vi "test report.vi"(6 "append report?":bool=TRUE, 7 "report path":path=path "C:/Users/andreika/Documents/work/SPELS_TEST/stm_test/TestReport.xlsx", 8 "error in":errorcluster, 9 "MS Office parameters in":T1, 10 "report in":refnum<class "NI_report.lvclass">, 11 "test data cluster":T2 {"elements 2" format="%x"; "elements 1" format="%x"}) -> (0 "error out":errorcluster, 1 "report path out":path, 2 "MS Office parameters out":T1, 3 "report out":refnum<class "NI_report.lvclass">)   [LabVIEW 2017, in "SPELS test.lvlib"]
uses:
  SPELS test.lvlib
  <vilib>/Utility/NIReport.llb/NI_report.lvclass
  <vilib>/Utility/NIReport.llb/Append Report Text (str wrap).vi
  <vilib>/Utility/NIReport.llb/Excel/NI_Excel.lvclass
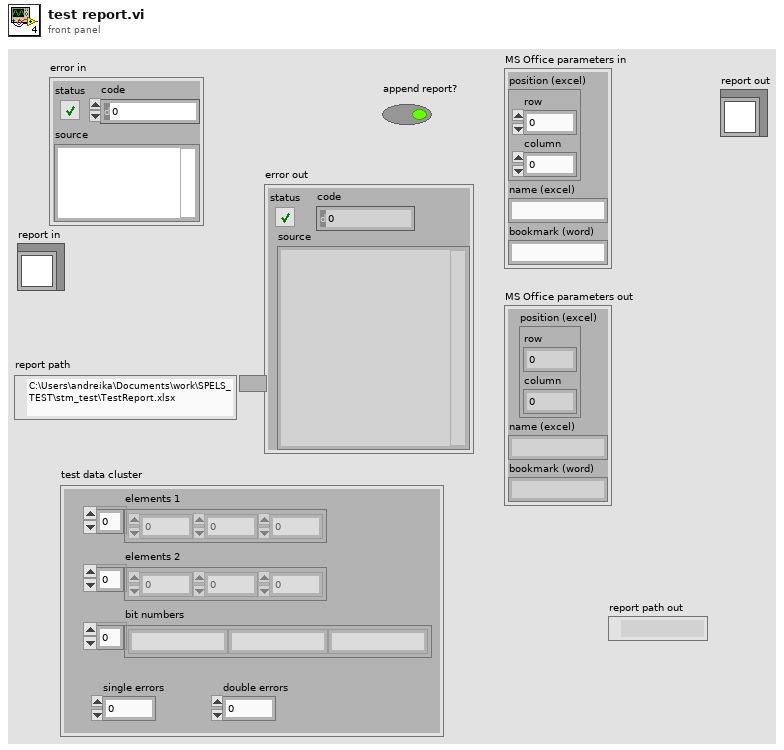
[diagram p1: front panel]
types:
  T1 = cluster{"position (excel)":cluster{"row":i32, "column":i32}, "name (excel)":string, "bookmark (word)":string}
  T2 = cluster{"elements 1 ":u8[], "elements 2":u8[], "bit numbers":string[], "single errors":u8, "double errors":u8}
  T3 = enum16{"Standard Report", "HTML", "Word", "Excel"}
  T4 = enum16{"maximized", "minimized", "normal", "no change"}
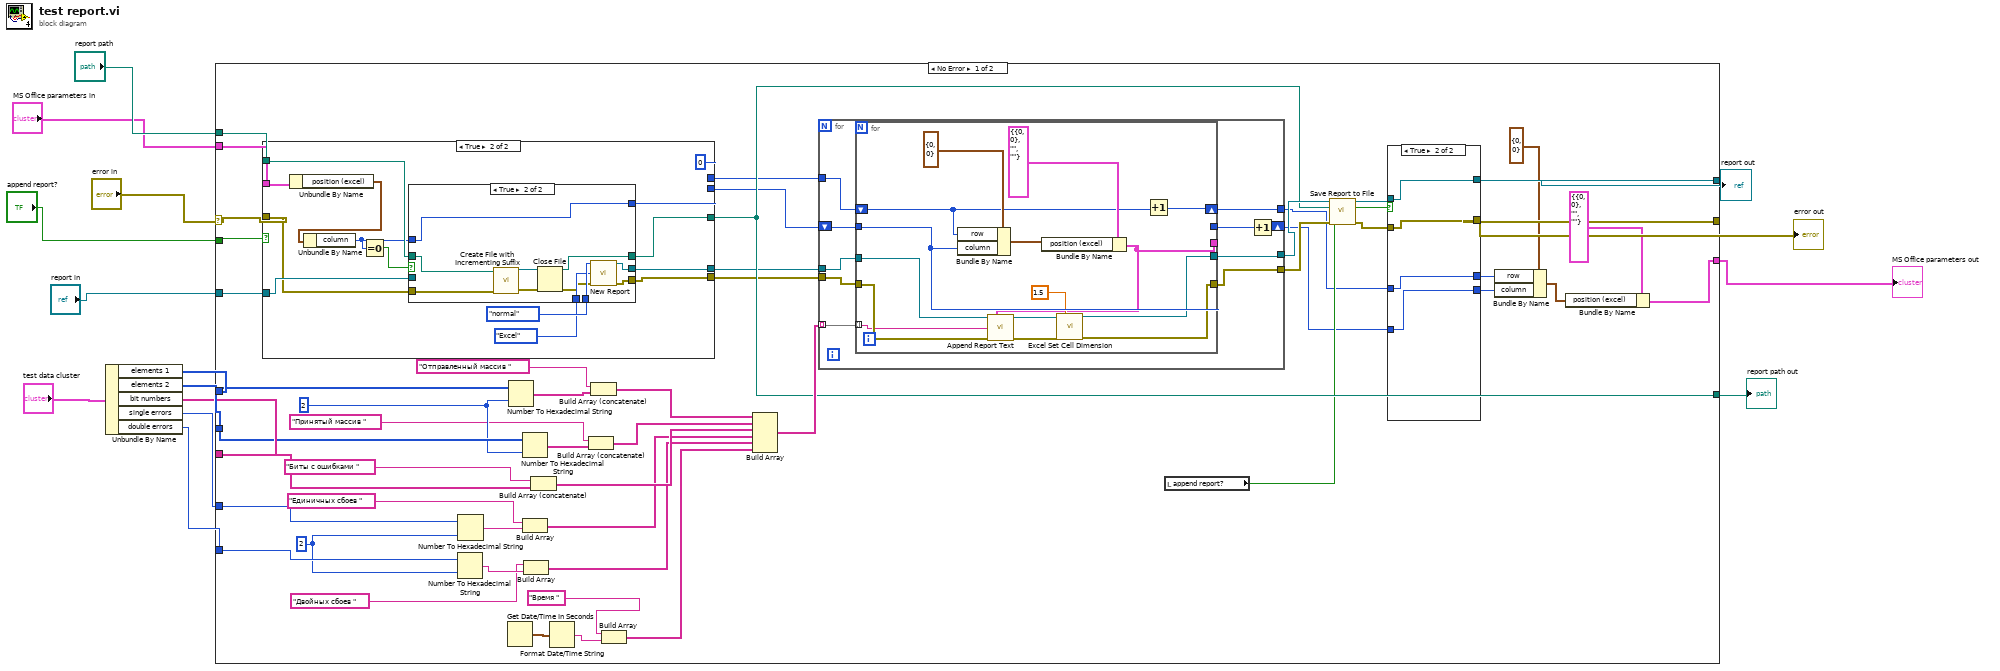
[diagram p0: block diagram]
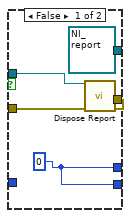
[diagram p2: hidden frame]
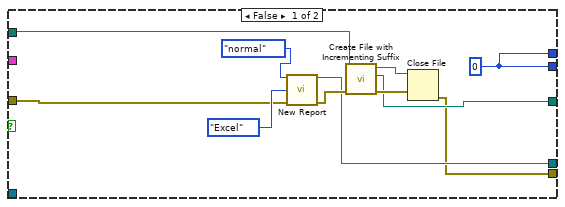
[diagram p3: hidden frame]
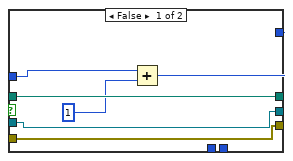
[diagram p4: hidden frame]
diagram:
  n1 = Unbundle By Name("test data cluster") -> ("elements 1"=w10:u8[], "elements 2"=w9:u8[], "bit numbers"=w8:string[], "single errors"=w7:u8, "double errors"=w6:u8)
  n2 = case shown="No Error" "error in" {
    selector: "error in" -> [w64 w146]
    tunnel: [w26 w146] -> w14
    tunnel: "append report?" -> [w66 _]
    tunnel: "report path" -> [w63 w144]
    tunnel: w10 -> [w62 _]
    tunnel: w9 -> [w61 _]
    tunnel: w8 -> [w55 _]
    tunnel: w7 -> [w46 _]
    tunnel: w6 -> [w47 _]
    tunnel: [w18 w145] -> w5
    tunnel: "MS Office parameters in" -> [w35 w145]
    tunnel: [w34 w144] -> w3
    tunnel: "report in" -> [w29 w143]
    tunnel: [w25 w143] -> w1
    frame No Error {
      w45 = i16 2 ("width (-)")
      w60 = i16 2 ("width (-)")
      n3 = case shown="True" w66 {
        tunnel: w64 -> [w109 w115]
        tunnel: w63 -> [w108 w114]
        tunnel: [w104 w124] -> w34
        tunnel: w35 -> [_ w125]
        tunnel: [w103 0] -> w33
        tunnel: [w103 w122] -> w32
        tunnel: [w102 w118] -> w31
        tunnel: [w101 w116] -> w30
        tunnel: w29 -> [_ w117]
        frame False {
          w103 = 0 ("row")
          n4 = call <vilib>:"New Report.vi"("window state (normal)"=T4."normal", "report type"=T3."Excel", "error in (no error)"=w109) -> ("report out"=w102:refnum<class "NI_report.lvclass">, "error out"=w107:errorcluster)  [unwired: 11 in]
          n5 = call <vilib>:"Create File with Incrementing Suffix.vi"("error in (no error)"=w107, "file path"=w108) -> ("error out"=w105:errorcluster, "actual path"=w104:path, "refnum out"=w106:refnum<file>)  [unwired: 7 in]
          n6 = Close File(refnum=w106, error in=w105) -> (error out=w101:errorcluster)  [unwired: 1 out]
        }
        frame True {
          n7 = Unbundle By Name(w125) -> ("position (excel)"=w123:cluster{"row":i32, "column":i32})
          n8 = Unbundle By Name(w123) -> ("column"=w113:i32)
          n9 = Equal To 0?(x=w113) -> (x = 0?=w112:bool)
          n10 = case shown="True" w112 {
            tunnel: w114 -> [w131 w136]
            tunnel: w115 -> [w126 w135]
            tunnel: [w126 w137] -> w116
            tunnel: [w131 w142] -> w124
            tunnel: w113 -> [w128 w132]
            tunnel: [w129 w132] -> w122
            tunnel: T4."normal" ("window state (normal)") -> [_ w141]
            tunnel: T3."Excel" ("report type") -> [_ w140]
            tunnel: [w127 w138] -> w118
            tunnel: w117 -> [w127 _]
            frame False {
              n11 = Add(x=w128, y=1) -> (x+y=w129:i32)
            }
            frame True {
              n12 = call <vilib>:"Create File with Incrementing Suffix.vi"("error in (no error)"=w135, "file path"=w136) -> ("error out"=w134:errorcluster, "refnum out"=w133:refnum<file>)  [unwired: 7 in, 1 out]
              n13 = Close File(refnum=w133, error in=w134) -> (path=w142:path, error out=w139:errorcluster)
              n14 = call <vilib>:"New Report.vi"("window state (normal)"=w141, "report type"=w140, "error in (no error)"=w139) -> ("report out"=w138:refnum<class "NI_report.lvclass">, "error out"=w137:errorcluster)  [unwired: 11 in]
            }
          }
        }
      }
      n15 = Number To Hexadecimal String(1:w45, 2:w47) -> (0:w42:string)
      n16 = Number To Hexadecimal String(1:w45, 2:w46) -> (0:w44:string)
      n17 = Get Date/Time In Seconds() -> (seconds since 1Jan1904=w65:timestamp)
      n18 = Number To Hexadecimal String(1:w60, 2:w62) -> (0:w59:string[])
      n19 = Number To Hexadecimal String(1:w60, 2:w61) -> (0:w57:string[])
      n20 = Build Array("Единичных сбоев ", w44) -> (w40:string[])
      n21 = Build Array("Двойных сбоев ", w42) -> (w39:string[])
      n22 = Build Array (concatenate)("Биты с ошибками ", w55) -> (w53:string[])
      n23 = Format Date/Time String(seconds (now)=w65) -> (date/time string=w38:string)  [unwired: 2 in]
      n24 = Build Array (concatenate)("Принятый массив ", w57) -> (w52:string[])
      n25 = Build Array (concatenate)("Отправленный массив ", w59) -> (w51:string[])
      n26 = Build Array("Время ", w38) -> (w36:string[])
      n27 = Build Array(w51, w52, w53, w40, w39, w36) -> (w50:string[][])
      n28 = for {
        tunnel: [w85] -> w49
        tunnel: w50 -> [w81] mode=indexing
        shift-right: [w84] -> w23
        shift-left: w32 -> [w83]
        tunnel: [w80] -> w48
        tunnel: w33 -> [w79]
        tunnel: w31 -> [w78]
        tunnel: w30 -> [w77]
        tunnel: [w76] -> w22
        n29 = for {
          tunnel: w78 -> [w100]
          tunnel: w77 -> [w99]
          tunnel: [w88] -> w85
          shift-right: [w98] -> w76
          shift-left: w79 -> [w94]
          tunnel: w83 -> [w93]
          tunnel: [w93] -> w82
          tunnel: w81 -> [w92] mode=indexing
          tunnel: [w89] -> w80
          tunnel: [w86] -> _
          n30 = Bundle By Name(cluster=cluster{"row":i32, "column":i32} {"row"=0, "column"=0} ("position (excel)"), "row"=w94, "column"=w93) -> (w95:cluster{"row":i32, "column":i32})
          n31 = Bundle By Name(cluster=T1 {"position (excel)"={"row"=0, "column"=0}, "name (excel)"="", "bookmark (word)"=""} ("MS Office parameters"), "position (excel)"=w95) -> (w86:T1)
          n32 = call-poly <vilib>:"Append Report Text.vi"("report in"=w100, "MS Office parameters"=w86, "text"=w92, "error in (no error)"=w99) -> ("report out"=w91:refnum<class "NI_report.lvclass">, "error out"=w90:errorcluster)  [unwired: 8 in, 2 out]
          n33 = call <vilib>:"Excel Set Cell Dimension.vi"("report in"=w91, "width (-1)"=1.5, "error in (no error)"=w90) -> ("report out"=w89:refnum<class "NI_report.lvclass">, "error out"=w88:errorcluster)  [unwired: 11 in]
          n34 = Increment(x=w94) -> (x+1=w98:i32)
        }
        n35 = Increment(x=w82) -> (x+1=w84:i32)
      }
      n36 = local read "append report?"() -> (w24:bool)
      n37 = call-dynamic "Save Report to File.vi"("report in"=w48, "report file path"=w34, "error in (no error)"=w49) -> ("report out"=w27:refnum<class "NI_report.lvclass">, "error out"=w28:errorcluster)  [unwired: 11 in]
      n38 = case shown="True" w24 {
        tunnel: w28 -> [w71 w74]
        tunnel: w27 -> [w70 w75]
        tunnel: [w69 w74] -> w26
        tunnel: [refnum<class "NI_report.lvclass"> refnum ("report in") w75] -> w25
        tunnel: w23 -> [_ w72]
        tunnel: w22 -> [_ w73]
        tunnel: [w67 w73] -> w17
        tunnel: [w67 w72] -> w16
        frame False {
          w67 = 0
          n39 = call-dynamic "Dispose Report.vi"("report in"=w70, "error in (no error)"=w71) -> ("error out"=w69:errorcluster)  [unwired: 13 in]
        }
        frame True {
        }
      }
      n40 = Bundle By Name(cluster=cluster{"row":i32, "column":i32} {"row"=0, "column"=0} ("position (excel)"), "row"=w17, "column"=w16) -> (w21:cluster{"row":i32, "column":i32})
      n41 = Bundle By Name(cluster=T1 {"position (excel)"={"row"=0, "column"=0}, "name (excel)"="", "bookmark (word)"=""} ("MS Office parameters"), "position (excel)"=w21) -> (w18:T1)
    }
    frame Error {
    }
  }
  "error out" <- w14
  "MS Office parameters out" <- w5
  "report path out" <- w3
  "report out" <- w1
